vi "SRV_PM_Is Checksum Ok.vi"(0 "Packet Data":u8[](array[numeric]) format="%.0x", 9 "Total Packet Length":u16, 11 "error in (no error)":errorcluster, 12 "Gen Err? (T)":bool=TRUE) -> (8 "Checksum OK?":bool, 13 "Packet Data sans Extra Bytes":u8[](array[numeric]) format="%.0x", 14 "Extra Bytes":u8[](array[numeric]) format="%.0x", 15 "error out":errorcluster)   [LabVIEW 2014]
panel:
  out "Calculated Checksum":u8[](array[numeric]) format="%.0x"
  out "Stored Checksum":u8[](array[numeric]) format="%.0x"
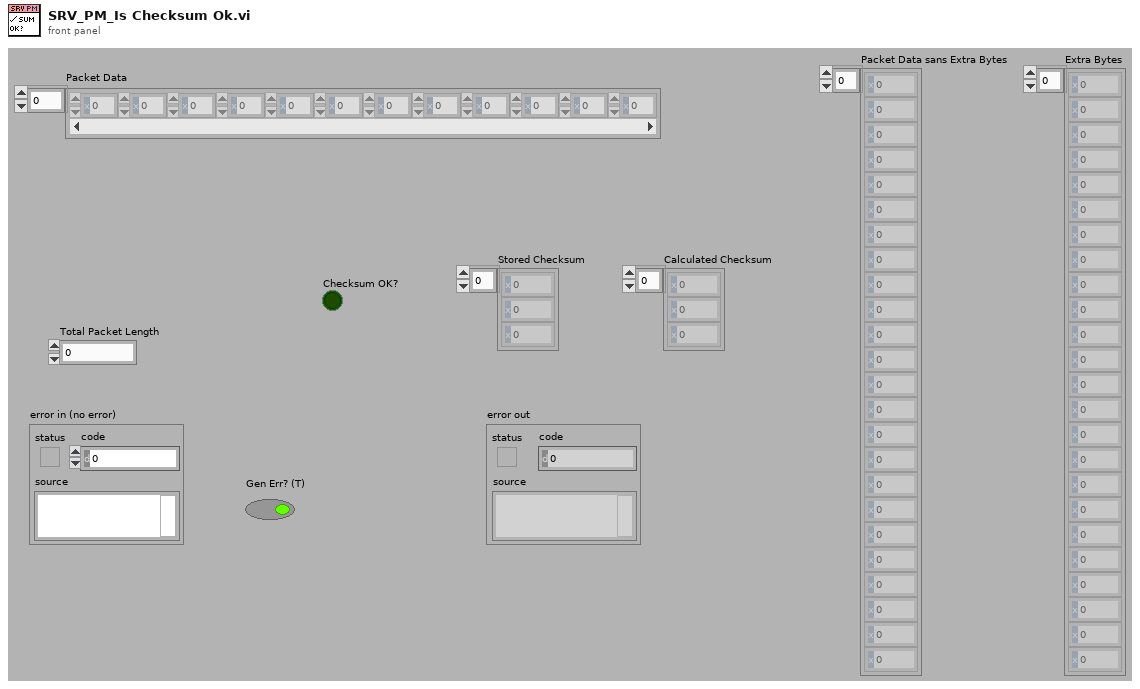
[diagram p1: front panel]
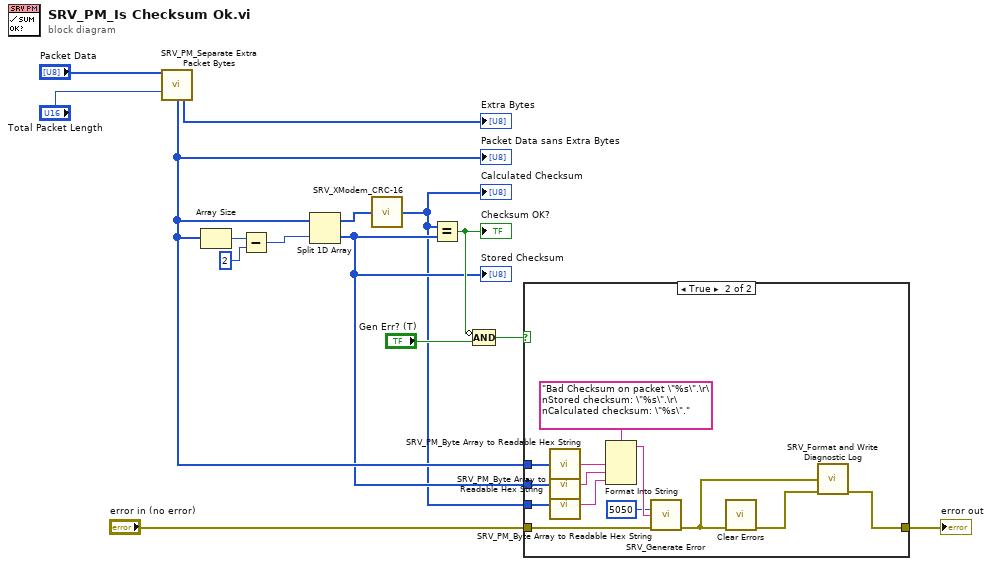
[diagram p0: block diagram]
diagram:
  n1 = call "SRV_PM_Separate Extra Packet Bytes.vi"("Packet"="Packet Data", "Total Packet Length"="Total Packet Length") -> ("Packet Data sans Extra Bytes"=w5:u8[], "Extra Bytes"=→"Extra Bytes":u8[])  [unwired: 11 in, 1 out]
  "Packet Data sans Extra Bytes" <- w5
  n2 = Array Size(array=w5) -> (size(s)=w15:i32)
  n3 = Subtract(x=w15, y=2) -> (x-y=w13:i32)
  n4 = Split 1D Array(array=w5, index=w13) -> (first subarray=w12:u8[], second subarray=w3:u8[])
  "Stored Checksum" <- w3
  n5 = call "SRV_XModem_CRC-16.vi"("Array"=w12) -> ("16-bit CRC Array"=w2:u8[])  [unwired: 14 in]
  "Calculated Checksum" <- w2
  n6 = Equal?(x=w2, y=w3) -> (x = y?=w11:bool)
  "Checksum OK?" <- w11
  n7 = Compound Arithmetic op=AND(invert w11, "Gen Err? (T)") -> (w9:bool)
  n8 = case shown="True" w9 {
    tunnel: w5 -> [_ w24]
    tunnel: "error in (no error)" -> [w16 w27]
    tunnel: [w16 w19] -> w7
    tunnel: w3 -> [_ w21]
    tunnel: w2 -> [_ w20]
    frame False {
    }
    frame True {
      n9 = call "SRV_PM_Byte Array to Readable Hex String.vi"("Byte Array"=w24) -> ("Readable Hex String"=w29:string)  [unwired: 14 in]
      n10 = call "SRV_PM_Byte Array to Readable Hex String.vi"("Byte Array"=w21) -> ("Readable Hex String"=w23:string)  [unwired: 14 in]
      n11 = call "SRV_PM_Byte Array to Readable Hex String.vi"("Byte Array"=w20) -> ("Readable Hex String"=w22:string)  [unwired: 14 in]
      n12 = Format Into String(format string="Bad Checksum on packet \"%s\".\r\nStored checksum: \"%s\".\r\nCalculated checksum: \"%s\"." ("Message"), w29, w23, w22) -> (resulting string=w28:string)  [unwired: 2 in, 1 out]
      n13 = call "SRV_Generate Error.vi"("code (42: generic error)"=5050, "Message"=w28, "error in (no error)"=w27) -> ("error out"=w18:errorcluster)  [unwired: 12 in]
      n14 = call <vilib>:"Clear Errors.vi"("error in (no error)"=w18) -> ("error out"=w17:errorcluster)  [unwired: 5 in, 1 out]
      n15 = call "SRV_Format and Write Diagnostic Log.vi"("error to log"=w18, "error in (no error)"=w17) -> ("error out"=w19:errorcluster)  [unwired: 13 in]
    }
  }
  "error out" <- w7
